vi "Format CSV Time Data.vi"(0 "Data_In":dbl[](array[numeric]) min=-200.0 max=50.0) -> (4 "Data_out":string)   [LabVIEW 2020, in "Anritsu Signal Analyzer Series.lvlib"]
doc: "Format Time Data(Double) to CSV Data String"
uses:
  Anritsu Signal Analyzer Series.lvlib
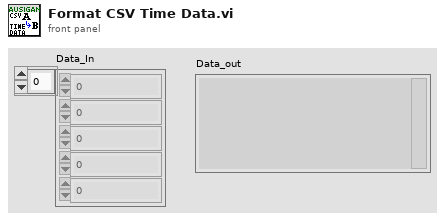
[diagram p1: front panel]
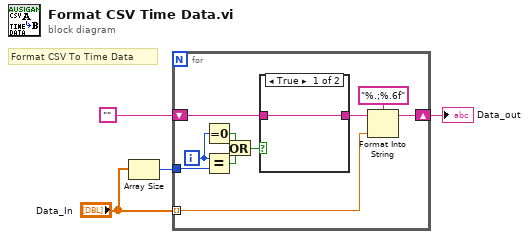
[diagram p0: block diagram]
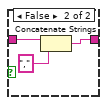
[diagram p2: hidden frame]
diagram:
  # "Format CSV To Time Data"
  n1 = Array Size(array="Data_In") -> (size(s)=w1:i32)
  n2 = for {
    shift-right: [w11] -> w3
    shift-left: "" -> [w14]
    tunnel: "Data_In" -> [w5] mode=indexing
    tunnel: w1 -> [w10]
    i -> [w6]
    n3 = Equal To 0?(x=w6) -> (x = 0?=w9:bool)
    n4 = Equal?(x=w6, y=w10) -> (x = y?=w8:bool)
    n5 = Or(x=w9, y=w8) -> (x .or. y?=w7:bool)
    n6 = case shown="True" w7 {
      tunnel: w14 -> [w15 w18]
      tunnel: [w15 w16] -> w13
      frame True {
      }
      frame False {
        n7 = Concatenate Strings(w18, "," ("string")) -> (w16:string)
      }
    }
    n8 = Format Into String(format string="%.;%.6f", initial string=w13, w5) -> (resulting string=w11:string)  [unwired: 1 in, 1 out]
  }
  "Data_out" <- w3
